vi "ExponentialFit0to60.vi"(11 "voltage":dbl) -> (3 "angle":dbl)   [LabVIEW 2022 SP3]
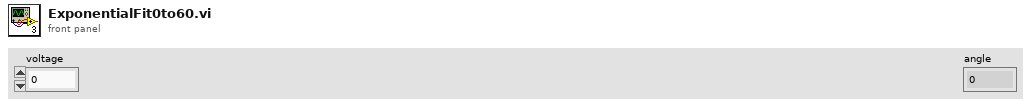
[diagram p1: front panel]
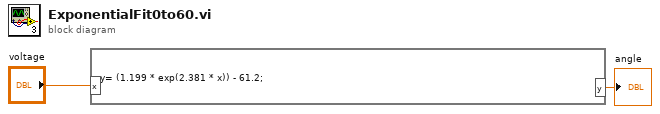
[diagram p0: block diagram]
diagram:
  n1 = formula code="y= (1.199 * exp(2.381 * x)) - 61.2;"("x"="voltage") -> ("y"=→"angle":dbl)
